vi "Read Count.vi"(8 "error in (no error)":errorcluster, 9 "Data Point Index (0: Last)":u16, 10 "Read B? (F)":bool, 11 "VISA resource name":refnum<visa-resource-name>) -> (0 "error out":errorcluster, 2 "Count":i16, 3 "VISA resource name out":refnum<visa-resource-name>)   [LabVIEW 2013, in "SRS SR400.lvlib"]
doc: "<B>QA { m }</B>\n<B>QB { m }</B>\n\nThe QA command reads the most recent complete data point from counter A, QB reads the most recent data point from counter B. QA and QB commands should only be sent after checking the Data Ready status bit. This bit is set at the end of each complete count period and signals the availability of valid data. The Data Ready status bit is reset after it is read. Sending QA or QB commands without polling the Data Ready status can cause data points to be read multiple times. Note that QA and QB do not reset the Data Ready status.\n\nIf data is not ready, the QA and QB commands return -1. If counter B is preset, QB returns -1.\n\nWhen m is included in a QA or QB command, buffered data from scan point m is read. m = 1 is the first data point in the scan and m = N PERIODS is the last data point. If m>2000 or m=0, an error occurs. If counter B is preset, then QB m returns 1.\n\nIf m > last completed point of the current scan, then -1 is returned. Therefore during a scan, QA 1 can be sent until a positive count is returned. At this point, the QA 2 command should be sent until a positive count is returned. All data from the scan can be read in this manner. This is the fastest way to read data during a scan while still maintaining full handshaking.\n\nData from the scan buffer can also be read after the scan is completed. The Scan Done status bit can be polled to determine when the scan finishes. The Scan Done status bit is set at the end of a scan only if the scan end mode is STOP. The Scan Done status bit is reset after it is read. To prevent ambiguity, the status byte should be cleared before starting a scan and then polled to determine when the scan is finished.\n\nWhenever scan data is to be read, the scan end mode should be STOP and a new scan started only after reading the desired data from the previous scan.\n\nIf m is absent or between 1 and 2000, data is always returned from a Q command. The value -1 is reserved for errors."
uses:
  <instrlib>/SRS SR400/SRS SR400.lvlib
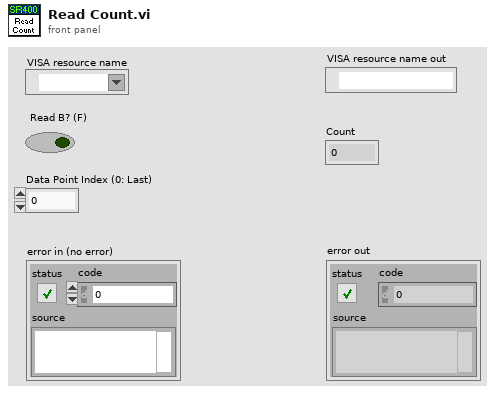
[diagram p1: front panel]
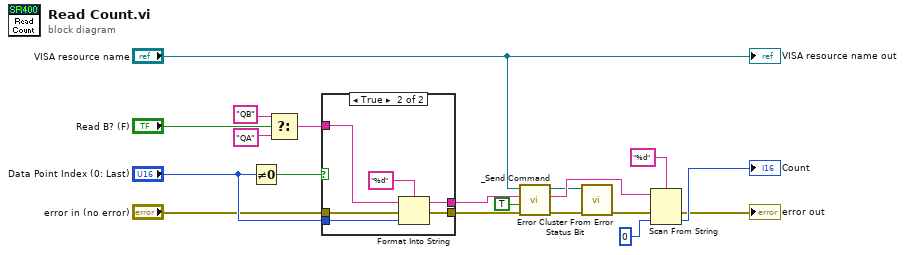
[diagram p0: block diagram]
diagram:
  n1 = Not Equal To 0?(x="Data Point Index (0: Last)") -> (x != 0?=w6:bool)
  n2 = Select(t="QB" ("command"), s="Read B? (F)", f="QA" ("command")) -> (s? t:f=w5:string)
  n3 = case shown="True" w6 {
    tunnel: "Data Point Index (0: Last)" -> [_ w27]
    tunnel: w5 -> [w21 w25]
    tunnel: [w21 w24] -> w4
    tunnel: [w20 w22] -> w1
    tunnel: "error in (no error)" -> [w20 w23]
    frame False {
    }
    frame True {
      n4 = Format Into String(format string="%d", initial string=w25, error in=w23, w27) -> (resulting string=w24:string, error out=w22:errorcluster)
    }
  }
  n5 = call <instrlib>:"_Send Command.vi"("error in (no error)"=w1, "Read Value? (F)"=TRUE, "Command"=w4, "VISA resource name"="VISA resource name") -> ("error out"=w11:errorcluster, "Response"=w9:string, "VISA resource name out"=w8:refnum<visa-resource-name>)  [unwired: 5 out]
  n6 = call <instrlib>:"Error Cluster From Error Status Bit.vi"("error in (no error)"=w11, "VISA resource name"=w8) -> ("error out"=w10:errorcluster)  [unwired: 8 in, 1 out]
  n7 = Scan From String(format string="%d", input string=w9, error in=w10, default 1=i16 0 ("default value 1")) -> (error out=→"error out":errorcluster, output 1=→"Count":i16)  [unwired: 1 in, 2 out]
  "VISA resource name out" <- "VISA resource name"
